vi "VelocityProfileMove.vi"(8 "error in (no error)":errorcluster, 10 "Array":dbl[](array[numeric]), 11 "SoftmotionAxis in":refnum<class "SoftmotionAxis.lvclass">) -> (0 "error out":errorcluster, 3 "SoftmotionAxis out":refnum<class "SoftmotionAxis.lvclass">)   [LabVIEW 2017, in "SoftmotionAxis.lvclass"]
uses:
  SoftmotionAxis.lvclass
  <resource>/objmgr/nimotion.rc
  Utilities/WordManipulationLibrary.lvlib
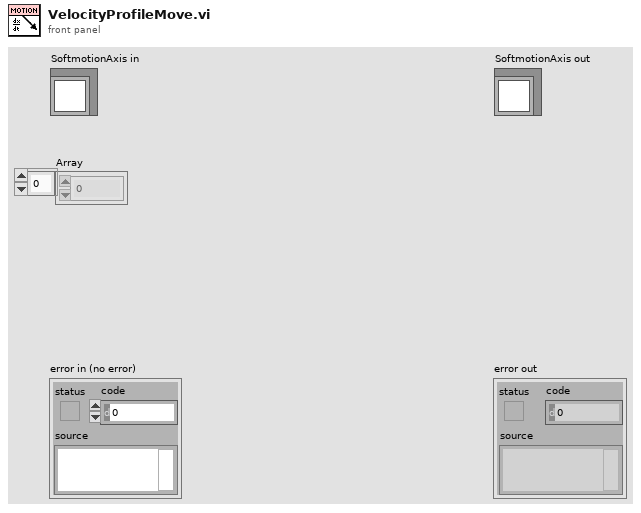
[diagram p1: front panel]
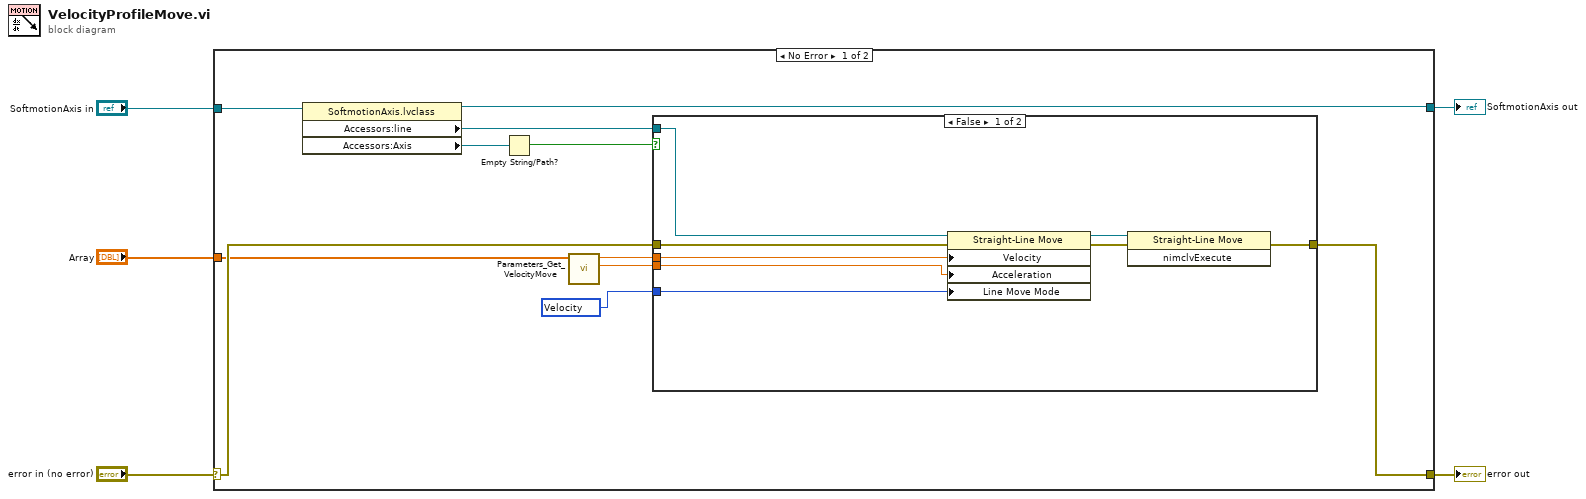
[diagram p0: block diagram]
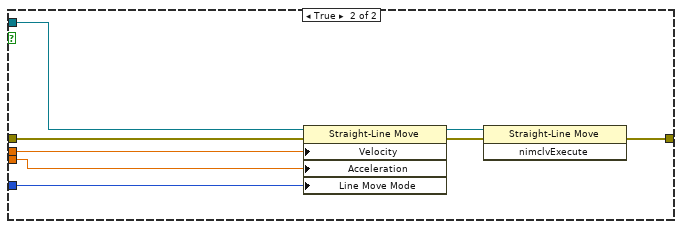
[diagram p2: hidden frame]
diagram:
  n1 = case shown="No Error" "error in (no error)" {
    selector: "error in (no error)" -> [w10 w34]
    tunnel: [w16 w34] -> w4
    tunnel: [w14 w33] -> w2
    tunnel: "SoftmotionAxis in" -> [w15 w33]
    tunnel: "Array" -> [w8 _]
    frame No Error {
      w9 = 10551346 items=["Relative"=10551344, "Absolute"=10551337, "Relative To Capture"=10551345, "Velocity"=10551346, "Polyline"=11600101] ("Line Move Mode")
      n2 = property class="SoftmotionAxis.lvclass"(reference=w15) -> (reference out=w14:refnum<class "SoftmotionAxis.lvclass">, "Accessors:line"=w13:refnum<k20>, "Accessors:Axis"=w12:refnum<k21>)  [unwired: 1 in, 1 out]
      n3 = Empty String/Path?(string/path=w12) -> (empty?=w11:bool)
      n4 = call "Parameters_Get_VelocityMove.vi"("Parameters"=w8) -> ("Acceleration"=w6:dbl, "Velocity"=w7:dbl)  [unwired: 8 in, 1 out]
      n5 = case shown="False" w11 {
        tunnel: [w22 w30] -> w16
        tunnel: w13 -> [w21 w29]
        tunnel: w10 -> [w20 w28]
        tunnel: w9 -> [w19 w27]
        tunnel: w7 -> [w18 w26]
        tunnel: w6 -> [w17 w25]
        frame False {
          n6 = property class="Straight-Line Move"(reference=w21, error in=w20, "Velocity"=w18, "Acceleration"=w17, "Line Move Mode"=w19) -> (reference out=w23:refnum<k20>, error out=w24:errorcluster)
          n7 = invoke class="Straight-Line Move" method="nimclvExecute"(reference=w23, error in=w24) -> (error out=w22:errorcluster)  [unwired: 1 in, 2 out]
        }
        frame True {
          n8 = property class="Straight-Line Move"(reference=w29, error in=w28, "Velocity"=w26, "Acceleration"=w25, "Line Move Mode"=w27) -> (reference out=w31:refnum<k20>, error out=w32:errorcluster)
          n9 = invoke class="Straight-Line Move" method="nimclvExecute"(reference=w31, error in=w32) -> (error out=w30:errorcluster)  [unwired: 1 in, 2 out]
        }
      }
    }
    frame Error {
    }
  }
  "error out" <- w4
  "SoftmotionAxis out" <- w2
